vi "RSZVB Trace Add Mode.vi"(6 "In Mode (Single-ended)":i32(ring) items=["Single-ended", "Differential", "Common"], 7 "Out Mode (Single-ended)":i32(ring) items=["Single-ended", "Differential", "Common"], 8 "error in (no error)":errorcluster {"code" format="%.0x"}, 9 "Trace Name (\"Trc1\")":string="Trc1", 10 "Channel (1)":i32=1, 11 "VISA session":refnum<visa-resource-name>) -> (0 "error out":errorcluster {"code" format="%.0x"}, 3 "dup VISA session":refnum<visa-resource-name>)   [LabVIEW 2011]
doc: "This VI creates a new trace in the current diagram area and assigns it to the selected channel. The new trace is created with the default trace and channel settings. Trace is not displayed. \n\nRemote-control command(s):\nCALCulate<Ch>:PARameter:SDEFine"
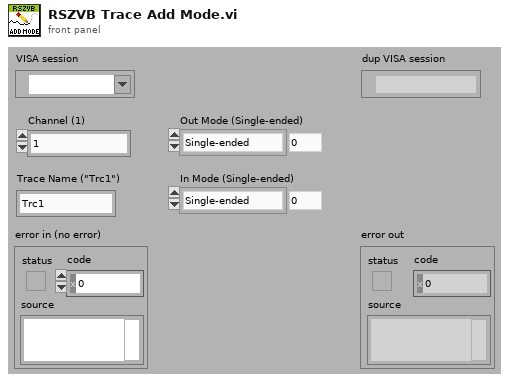
[diagram p1: front panel]
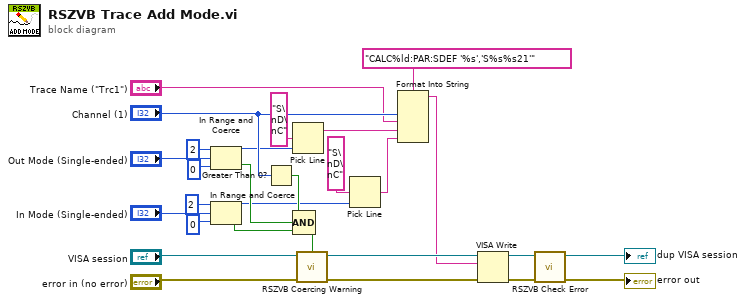
[diagram p0: block diagram]
diagram:
  n1 = In Range and Coerce(upper limit=2 ("lower limit"), x="Out Mode (Single-ended)", lower limit=0) -> (coerced(x)=w8:i32, In Range?=w6:bool)
  n2 = In Range and Coerce(upper limit=2 ("lower limit"), x="In Mode (Single-ended)", lower limit=0) -> (coerced(x)=w3:i32, In Range?=w5:bool)
  n3 = Greater Than 0?(x="Channel (1)") -> (x > 0?=w22:bool)
  n4 = Pick Line(multi-line string="S\nD\nC", line index=w8) -> (output string=w1:string)  [unwired: 1 in]
  n5 = Compound Arithmetic op=AND(w22, w6, w5) -> (w7:bool)
  n6 = call "RSZVB Coercing Warning.vi"("In Range?"=w7, "error in (no error)"="error in (no error)", "VISA session"="VISA session") -> ("error out"=w26:errorcluster, "dup VISA session"=w27:refnum<visa-resource-name>)  [unwired: 7 in]
  n7 = Pick Line(multi-line string="S\nD\nC", line index=w3) -> (output string=w2:string)  [unwired: 1 in]
  n8 = Format Into String(format string="CALC%ld:PAR:SDEF '%s','S%s%s21'", "Channel (1)", "Trace Name (\"Trc1\")", w1, w2) -> (resulting string=w23:string)  [unwired: 2 in, 1 out]
  n9 = VISA Write(VISA resource name=w27, write buffer=w23, error in (no error)=w26) -> (VISA resource name out=w24:refnum<visa-resource-name>, error out=w25:errorcluster)  [unwired: 1 out]
  n10 = call "RSZVB Check Error.vi"("error in (no error)"=w25, "VISA session"=w24) -> ("error out"=→"error out":errorcluster, "dup VISA session"=→"dup VISA session":refnum<visa-resource-name>)  [unwired: 8 in]
